vi "DeviceGlobals.vi"() -> ()   [LabVIEW 2020]
panel:
  out "ms timestamp network trigger":dbl
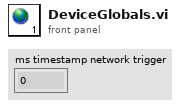
[diagram p1: front panel]
diagram:
